vi "Substitute Actor.vi"(10 "Substitute Actor in":refnum<class "Actor.lvclass">, 11 "Current Series Actor":refnum<class "Series Actor.lvclass">) -> (0 "error out":errorcluster, 2 "Substitute Actor out":refnum<class "Actor.lvclass">)   [LabVIEW 2024, in "Series Actor.lvlib" / "Series Actor.lvclass"]
doc: "(<B>Filename</B>: Actor Framework.lvlib:Actor.lvclass:Substitute Actor.vi)\n\nThis method copies information from the <b>Current Actor</b> to the <b>Substitute Actor</b>, including the to-self and the to-caller queue references. The purpose of this function is to allow an actor to define a method that replaces itself with another actor, useful for implementing a State Pattern Actor. Child classes should override this method to copy any additional fields that they need from the current to the substitute.\n\nThis method may return error code 678010: Illegal substitution. Overrides of this method may choose to return this error if the new actor is not one that is an appropriate substitute for the current actor, for whatever standards of \"appropriate\" are chosen for the current actor. If returning an error, override VIs should return the unmodified <b>Current Actor</b> as <b>Substitute Actor out</b>."
uses:
  Series Actor.lvclass
  Series Actor.lvclass/Series Actor.ctl
  <vilib>/ni/Actors/State Actor/State Actor/State Actor.lvclass
  C:/Program Files/National Instruments/LabVIEW 2024/vi.lib/ni/Actors/State Actor/State Actor/State Actor.lvclass
  C:/Program Files/National Instruments/LabVIEW 2024/vi.lib/ActorFramework/Actor/Actor.lvclass
  D:/git/HAL/MAL/Series/Series Actor/Series Actor/Series Actor.lvclass
  D:/git/HAL/MAL/Series/ISeries Actor/ISeries Actor/ISeries Actor.lvclass
  <vilib>/ActorFramework/Actor/Actor.lvclass
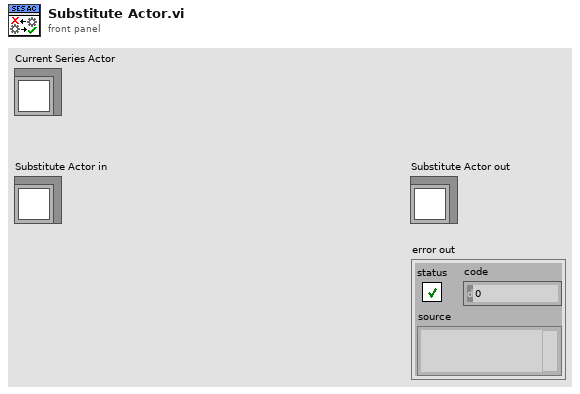
[diagram p1: front panel]
types:
  T1 = map{string, refnum<class "Message Enqueuer.lvclass">}
  T2 = map{enum16{""}, refnum<class "Message Enqueuer.lvclass">}
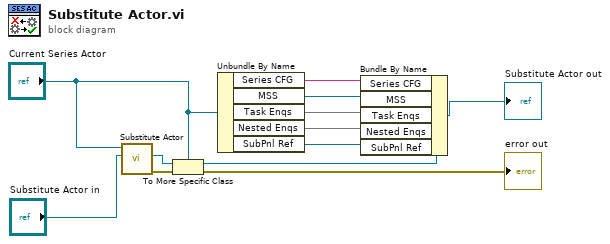
[diagram p0: block diagram]
diagram:
  n1 = call-parent "Substitute Actor.vi"("Substitute Actor in"="Substitute Actor in", "Current Actor"="Current Series Actor") -> ("error out"=w11:errorcluster, "Substitute Actor out"=w9:refnum<class "Actor.lvclass">)  [unwired: 8 in]
  n2 = To More Specific Class(target class="Current Series Actor", reference=w9, error in=w11) -> (specific class reference=w7:refnum<class "Series Actor.lvclass">, error out=→"error out":errorcluster)
  n3 = Unbundle By Name("Current Series Actor") -> ("Series CFG"=w5:string, "MSS"=w4:refnum<class "MSS.lvclass">, "Task Enqs"=w3:T1, "Nested Enqs"=w2:T2, "SubPnl Ref"=w1:refnum<vi>)
  n4 = Bundle By Name(cluster=w7, "Series CFG"=w5, "MSS"=w4, "Task Enqs"=w3, "Nested Enqs"=w2, "SubPnl Ref"=w1) -> (→"Substitute Actor out":refnum<class "Series Actor.lvclass">)
